vi "ex3.vi"(1 "Numeric 2":i32) -> (0 "Numeric":dbl)   [LabVIEW 2019]
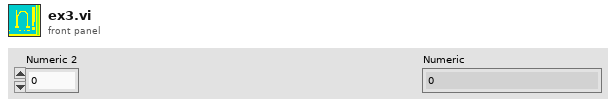
[diagram p1: front panel]
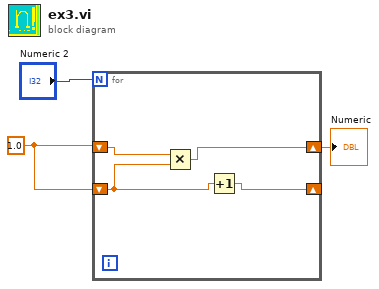
[diagram p0: block diagram]
diagram:
  w3 = 1.0
  n1 = for {
    N: "Numeric 2" -> [_]
    shift-right: [w6] -> w2
    shift-left: w3 -> [w7]
    shift-right: [w4] -> _
    shift-left: w3 -> [w5]
    n2 = Multiply(x=w7, y=w5) -> (x*y=w6:dbl)
    n3 = Increment(x=w5) -> (x+1=w4:dbl)
  }
  "Numeric" <- w2
